vi "New Boolean Evaluation Trigger.vi"(7 "Operand":T1, 8 "error in (no error)":errorcluster, 11 "Value":dbl) -> (0 "error out":errorcluster, 3 "Boolean Evaluation Trigger out":refnum<class "Boolean Evaluation Trigger.lvclass">)   [LabVIEW 2012, in "Waveform Data Logger Engine.lvlib" / "Boolean Evaluation Trigger.lvclass"]
uses:
  Boolean Evaluation Trigger.lvclass
  Operand.ctl
  Boolean Evaluation Trigger.lvclass/Boolean Evaluation Trigger.ctl
  Trigger/Trigger Type.ctl
  Trigger/Trigger.lvclass/Trigger.ctl
  Trigger/Write Trigger Type.vi
  Trigger/Trigger.lvclass
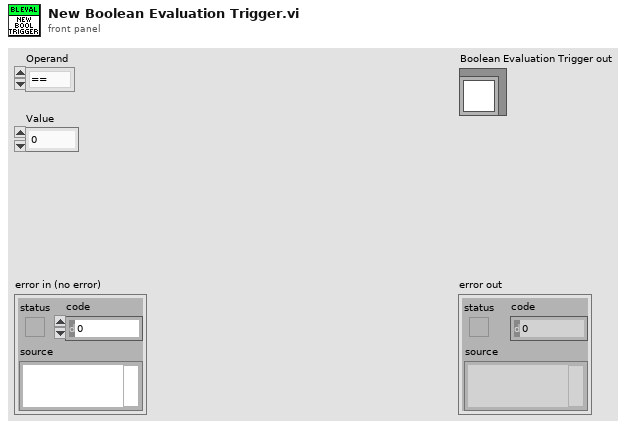
[diagram p1: front panel]
types:
  T1 = typedef "Waveform Data Logger Engine.lvlib/Boolean Evaluation Trigger.lvclass/Operand.ctl" = enum16{"==", "!=", "<", "<=", ">", ">="}
  T2 = typedef "Waveform Data Logger Engine.lvlib/Trigger.lvclass/Trigger Type.ctl" = enum16{"Default", "Digital Edge", "Analog Edge", "In Range", "Value Change", "Boolean Evaluation"}
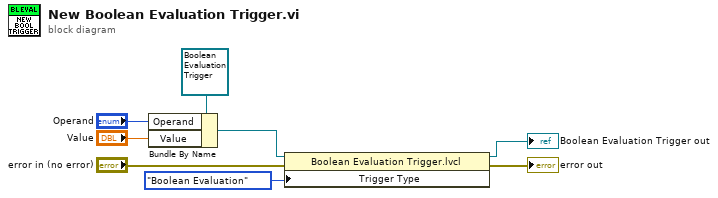
[diagram p0: block diagram]
diagram:
  n1 = Bundle By Name(cluster=refnum<class "Boolean Evaluation Trigger.lvclass"> refnum ("Boolean Evaluation Trigger in"), "Operand"="Operand", "Value"="Value") -> (w3:refnum<class "Boolean Evaluation Trigger.lvclass">)
  n2 = property class="Boolean Evaluation Trigger.lvcl"(reference=w3, error in="error in (no error)", "Trigger Type"=Trigger_Type."Boolean Evaluation") -> (reference out=→"Boolean Evaluation Trigger out":refnum<class "Boolean Evaluation Trigger.lvclass">, error out=→"error out":errorcluster)
